vi "Climb_Test.vi"(0 "B_Button":bool, 1 "Left_Joystick_Y":dbl, 2 "Y_Button":bool, 3 "Left_Joystick_Press":bool, 4 "Menu_Button":bool) -> ()   [LabVIEW 2018]
uses:
  Subsytems/Climb/Climb_Notifier.ctl
  Subsytems/Climb/Climb_Control_Type.ctl
  Global_Variables/Climb_Globals.vi
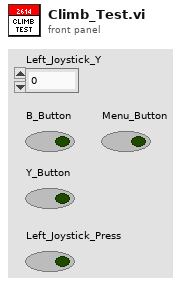
[diagram p1: front panel]
types:
  T1 = typedef "Climb_Notifier.ctl" = cluster{"Climb_Control_Type":T2, "Brake":bool, "Manual_Climb_Up":bool, "Manual_Drive_Forward":bool, "Manual_Drive_Backward":bool, "Manual_Climb_Down":bool, "Climb_Advance":bool, "Climb_Reverse":bool, "Parameter_One":dbl, "Parameter_Two":dbl, "Parameter_Three":dbl, "Step":i32, "Climb_Notifier":refnum<notifier>, "Climb_Distance":dbl, "Level_Two":bool, "Brake_State":bool, "Toggle_Servo":bool}
  T2 = typedef "Climb_Control_Type.ctl" = enum16{"No_Op", "Brake", "Manual_Climb_Up", "Manual_Climb_Down", "Manual_Drive_Forward", "Manual_Drive_Backward", "Back_Wheels_Forward", "Lift_Retract", "Lift_Extend", "Extend_to_Second_Level", "Spin"}
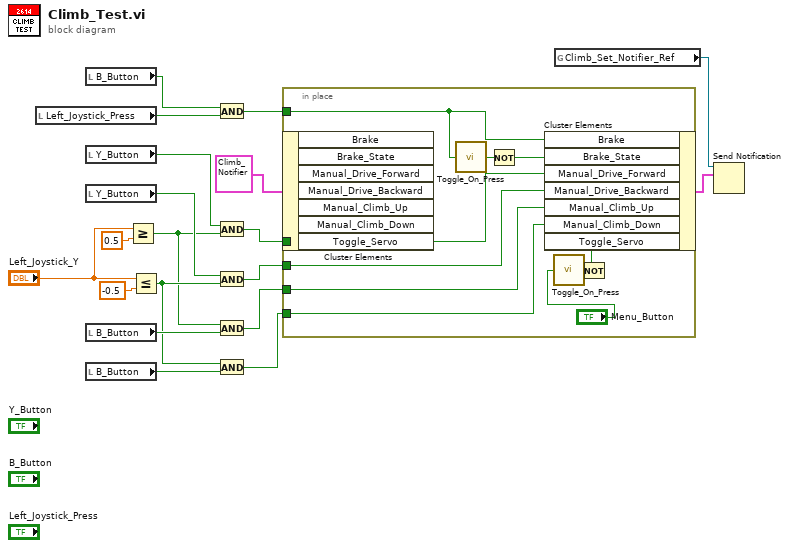
[diagram p0: block diagram]
diagram:
  n1 = local read "Left_Joystick_Press"() -> (w2:bool)
  n2 = local read "B_Button"() -> (w3:bool)
  n3 = local read "Y_Button"() -> (w13:bool)
  n4 = local read "Y_Button"() -> (w8:bool)
  n5 = local read "B_Button"() -> (w10:bool)
  n6 = local read "B_Button"() -> (w9:bool)
  n7 = Greater Or Equal?(x="Left_Joystick_Y", y=0.5) -> (x >= y?=w5:bool)
  n8 = Less Or Equal?(x="Left_Joystick_Y", y=-0.5) -> (x <= y?=w7:bool)
  n9 = And(x=w3, y=w2) -> (x .and. y?=w1:bool)
  n10 = And(x=w13, y=w5) -> (x .and. y?=w11:bool)
  n11 = And(x=w8, y=w7) -> (x .and. y?=w12:bool)
  n12 = And(x=w5, y=w10) -> (x .and. y?=w4:bool)
  n13 = And(x=w7, y=w9) -> (x .and. y?=w6:bool)
  n14 = in-place {
    in-place-border: w12 -> [w29]
    in-place-border: w11 -> [w28]
    in-place-border: w6 -> [w27]
    in-place-border: w4 -> [w26]
    in-place-border: w1 -> [w24]
    n15 = in-place-cluster #1(T1 {"Climb_Control_Type"=enum."No_Op", "Brake"=FALSE, "Manual_Climb_Up"=FALSE, "Manual_Drive_Forward"=FALSE, "Manual_Drive_Backward"=FALSE, "Manual_Climb_Down"=FALSE, "Climb_Advance"=FALSE, "Climb_Reverse"=FALSE, "Parameter_One"=0.0, "Parameter_Two"=0.0, "Parameter_Three"=0.0, "Step"=0, "Climb_Notifier"=refnum, "Climb_Distance"=0.0, "Level_Two"=FALSE, "Brake_State"=FALSE, "Toggle_Servo"=FALSE} ("Climb_Notifier")) -> ()  [unwired: 7 out]
    n16 = call "Toggle_On_Press.vi"("Boolean"=w24) -> ("Boolean Out"=w25:bool)
    n17 = Not(x=w25) -> (.not. x?=w23:bool)
    n18 = call "Toggle_On_Press.vi"("Boolean"="Menu_Button") -> ("Boolean Out"=w22:bool)
    n19 = Not(x=w22) -> (.not. x?=w21:bool)
    n20 = in-place-cluster #1("Brake"=w24, "Brake_State"=w23, "Manual_Drive_Forward"=w28, "Manual_Drive_Backward"=w29, "Manual_Climb_Up"=w26, "Manual_Climb_Down"=w27, "Toggle_Servo"=w21) -> (w19:T1)
  }
  n21 = global read "Climb_Globals.vi" "Climb_Set_Notifier_Ref"() -> (w17:refnum<notifier>)
  n22 = Send Notification(notification=w19, notifier=w17) -> ()  [unwired: 1 in, 2 out]
